vi "String Value Change.vi"(8 "New Value":string caption="新值", 9 "Display State In":T2 caption="显示状态输入", 11 "Include Paths Ref":refnum<vi> caption="包括路径引用") -> (1 "Display State Out":T2 caption="显示状态输出", 2 "Path Strings Out":T1 caption="路径字符串输出", 3 "Dup Include Paths Ref":refnum<vi> caption="包括路径引用副本")   [LabVIEW 2011, in "NISAST Include Paths.xctl"]
uses:
  NISAST Include Paths.xctl
  State.ctl
  Data.ctl
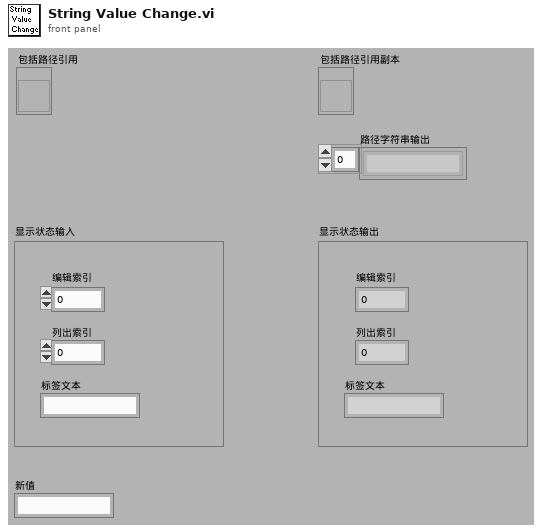
[diagram p1: front panel]
types:
  T1 = typedef "NISAST Include Paths.xctl/Data.ctl" = string[]
  T2 = typedef "NISAST Include Paths.xctl/State.ctl" = cluster{"Edit Index":i32, "List Index":i32, "Label Text":string}
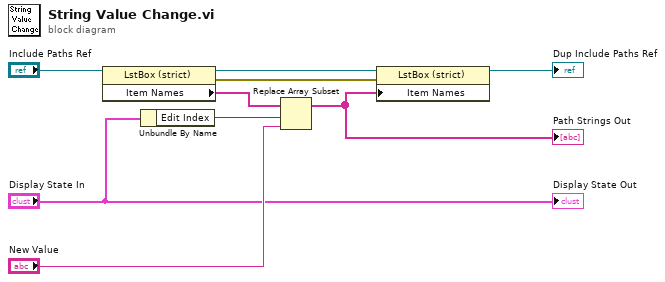
[diagram p0: block diagram]
diagram:
  n1 = property class="LstBox (strict)"(reference="Include Paths Ref") -> (reference out=w9:refnum<vi>, error out=w4:errorcluster, "Item Names"=w7:string[])  [unwired: 1 in]
  n2 = Unbundle By Name("Display State In") -> ("Edit Index"=w3:i32)
  n3 = Replace Array Subset(array=w7, new element="New Value", index=w3) -> (w2:string[])
  "Path Strings Out" <- w2
  n4 = property class="LstBox (strict)"(reference=w9, error in=w4, "Item Names"=w2) -> (reference out=→"Dup Include Paths Ref":refnum<vi>)  [unwired: 1 out]
  "Display State Out" <- "Display State In"
